vi "Rst.vi"(8 "Error":errorcluster caption="错误输入（无错误）", 10 "Timeout Value":u32=10000, 11 "VISA resource name":refnum<visa-resource-name>) -> (0 "Error out":errorcluster caption="错误输出", 3 "VISA resource name out":refnum<visa-resource-name>)   [LabVIEW 2020]
doc: "预设状态"
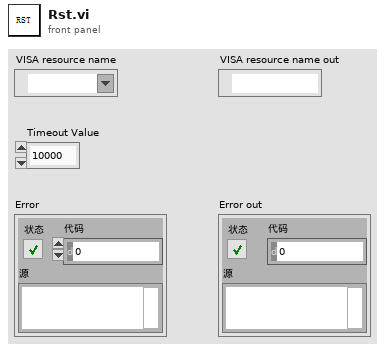
[diagram p1: front panel]
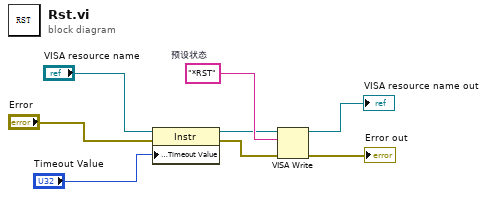
[diagram p0: block diagram]
diagram:
  w6 = "*RST"  # 预设状态
  n1 = property class="Instr"(reference="VISA resource name", error in="Error", "General Settings:Timeout Value"="Timeout Value") -> (reference out=w2:refnum<visa-resource-name>, error out=w1:errorcluster)
  n2 = VISA Write(VISA resource name=w2, write buffer=w6, error in (no error)=w1) -> (VISA resource name out=→"VISA resource name out":refnum<visa-resource-name>, error out=→"Error out":errorcluster)  [unwired: 1 out]
